vi "stoperaseLT_img.vi"   [LabVIEW 2015]
uses:
  phlib.dll
types:
  T1 = cluster{"initialized":bool, "devidx":i32, "Ch0 Level":i32, "Ch0 ZeroX":i32, "Ch1 Level":i32, "Ch1 ZeroX":i32, "sync rate":i32, "resolution":i32, "acq time":i32, "acq rate":i32, "# bins":u32, "Bin size":enum16{"1", "2", "4", "8", "16", "32", "64", "128"}, "min photons":u32, "truncate":u32}
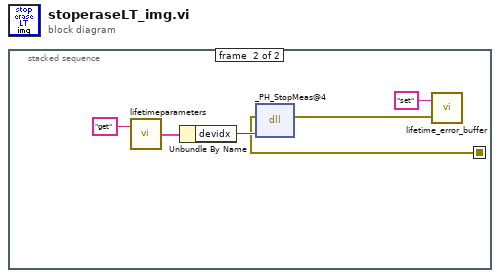
[diagram p0: block diagram]
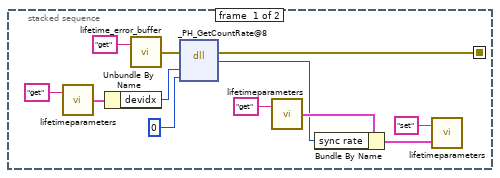
[diagram p2: hidden frame]
diagram:
  n1 = stacked-sequence {
    seq-local: [w1 _] -> [_ w13]
    frame #0 {
      n2 = call "lifetimeparameters.vi"("command"="get") -> ("Params out"=w5:T1)  [unwired: 1 in]
      n3 = Unbundle By Name(w5) -> ("devidx"=w4:i32)
      n4 = call "lifetime_error_buffer.vi"("command"="get") -> ("error out"=w2:errorcluster)  [unwired: 1 in]
      n5 = dll-call lib="phlib.dll" fn="_PH_GetCountRate@8" label="PH_GetCountRate"(error in=w2, "devidx"=w4, "channel"=0) -> (error out=w1:errorcluster, w7:i32)  [unwired: 4 in, 1 out]
      n6 = call "lifetimeparameters.vi"("command"="get") -> ("Params out"=w9:T1)  [unwired: 1 in]
      n7 = Bundle By Name(cluster=w9, "sync rate"=w7) -> (w8:T1)
      n8 = call "lifetimeparameters.vi"("Params in"=w8, "command"="set") -> ()  [unwired: 1 out]
    }
    frame #1 {
      n9 = call "lifetimeparameters.vi"("command"="get") -> ("Params out"=w15:T1)  [unwired: 1 in]
      n10 = Unbundle By Name(w15) -> ("devidx"=w14:i32)
      n11 = dll-call lib="phlib.dll" fn="_PH_StopMeas@4" label="PH_StopMeas"(error in=w13, "devidx"=w14) -> (error out=w17:errorcluster)  [unwired: 4 in, 1 out]
      n12 = call "lifetime_error_buffer.vi"("error in"=w17, "command"="set") -> ()  [unwired: 1 out]
    }
  }
